vi "Handle setConfiguration.vi"(8 "error in (no error)":errorcluster, 10 "setConfiguration":variant, 11 "Instrument.Template in":refnum<class "Instrument.Framework-Template.lvclass">) -> (0 "error out":errorcluster, 3 "Instrument.Template out":refnum<class "Instrument.Framework-Template.lvclass">)   [LabVIEW 2019, in "Instrument.Framework-Template.lvclass"]
uses:
  Instrument.Framework-Template.lvclass
  Instrument.Framework-Template.lvclass/Instrument.Framework-Template.ctl
  027c7e6d-2801-4a42-a61c-edfdd76072f6.vi
  027c7e6d-2801-4a42-a61c-edfdd76072f6.vi/1f6d7026-b9dc-41b4-a6b7-7f1bc59ea449.vi
  027c7e6d-2801-4a42-a61c-edfdd76072f6.vi/abc7ed59-e0d8-4e60-9620-0c326b0308e8.vi
  <vilib>/Utility/Data Type/Get Type Information.vi
  <vilib>/JDP Science/JSONtext/JSON text to Variant.vi
  <vilib>/JDP Science/JSONtext/LVClass Serializer/JSONtext LVClass Serializer.lvclass
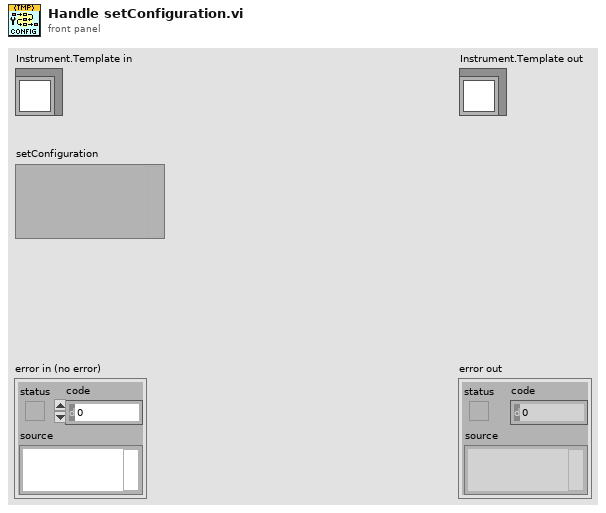
[diagram p1: front panel]
types:
  T1 = typedef "Instrument.Framework-Template.lvclass/Instrument.Framework-Template.Configuration--Cluster.ctl" = cluster{"Example Setting 1":dbl, "Example Setting 2":dbl, "Example Setting 3":string}
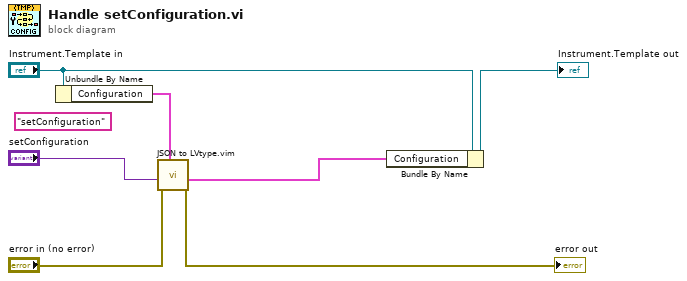
[diagram p0: block diagram]
diagram:
  (unwired) "setConfiguration" ("Command")
  n1 = Unbundle By Name("Instrument.Template in") -> ("Configuration"=w5:T1)
  n2 = call "JSON to LVtype.vim"("type"=w5, "error in (no error)"="error in (no error)", "JSON Data in"="setConfiguration") -> ("error out"=→"error out":errorcluster, "Data out"=w3:T1)  [unwired: 7 in]
  n3 = Bundle By Name(cluster="Instrument.Template in", "Configuration"=w3) -> (→"Instrument.Template out":refnum<class "Instrument.Framework-Template.lvclass">)
